vi "Draw ROI (user interactive).vi"(0 "Image file path":path) -> (1 "ROI to crop (pixels)":T1={"Xmax"=2147483647, "Ymax"=2147483647, "Xmin"=0, "Ymin"=0}, 2 "Error out":errorcluster)   [LabVIEW 2015]
doc: "Use this VI to mark a region-of-interest rectangle on an image, then programmatically output the ROI cluster and save the image with \"_ROI\" appended to current filename."
uses:
  Feature detection/Typedefs/ROI bounds.ctl
panel:
  in  "Quality":u32=750 max=1000
  out "Image showing ROI":T2(plugin-control)
  # "PN 04/04/2016"
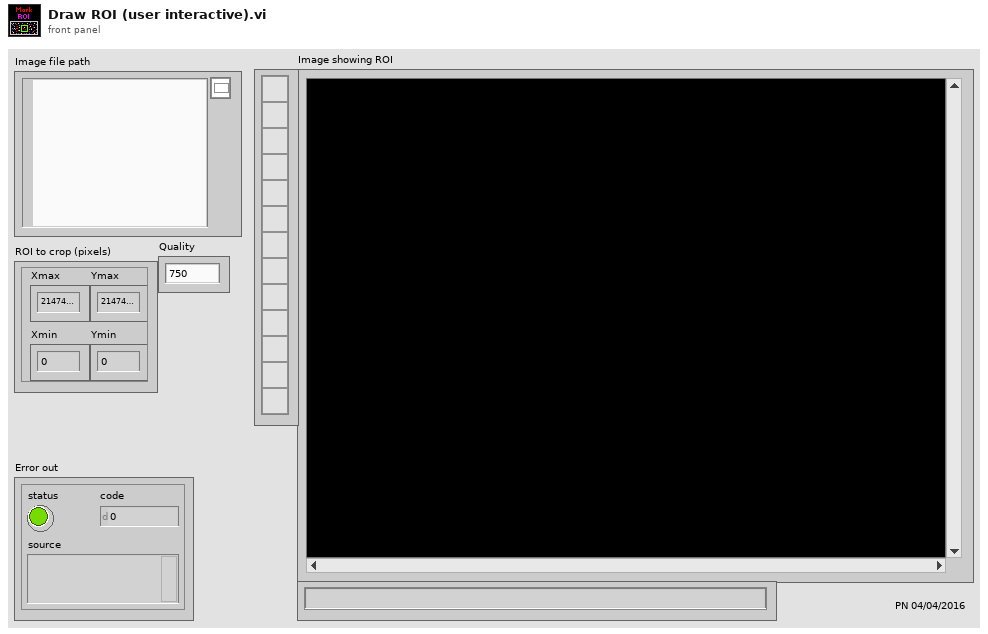
[diagram p1: front panel]
types:
  T1 = typedef "ROI bounds.ctl" = cluster{"Xmax":i32, "Ymax":i32, "Xmin":i32, "Ymin":i32}
  T2 = typedef "IMAQ Image.ctl" = refnum<image>
  T3 = cluster{"Left":i32, "Top":i32, "Right":i32, "Bottom":i32}
  T4 = typedef "Image Type" = u32
  T5 = typedef "IMAQ Rectangle" = cluster{"Left":i32, "Top":i32, "Right":i32, "Bottom":i32, "Rotation":dbl}
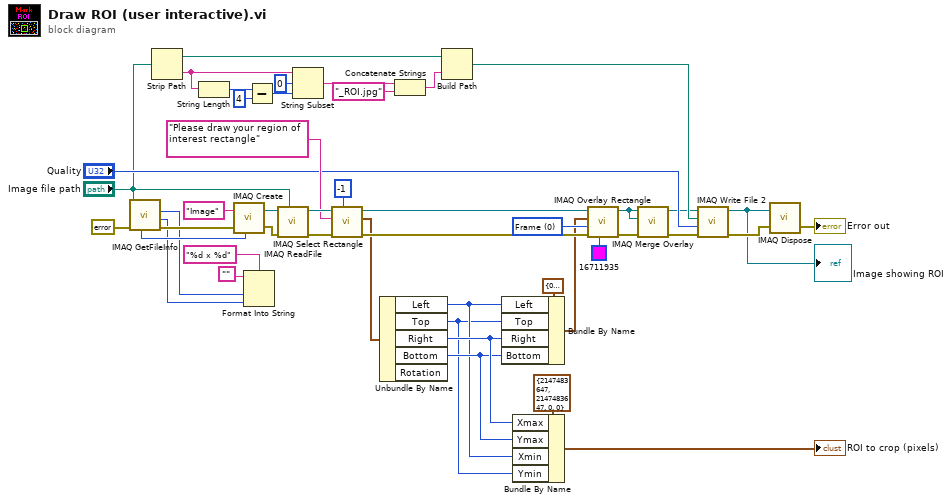
[diagram p0: block diagram]
diagram:
  w30 = u32 0 items=["Frame", "Fill", "Highlight"] ("Drawing Mode (Frame)")
  n1 = call "IMAQ GetFileInfo"("error in (no error)"=errorcluster {"status"=FALSE, "code"=0, "source"=""} ("error in"), "File Path"="Image file path") -> ("error out"=w41:errorcluster, "Y Resolution"=w39:i32, "X Resolution"=w40:i32, "Image Type"=w42:T4)  [unwired: 3 in, 3 out]
  n2 = Strip Path(path="Image file path") -> (stripped path=w14:path, name=w13:string)
  n3 = String Length(string=w13) -> (length=w12:i32)
  n4 = call "IMAQ Create"("Image Name"="Image", "Image Type"=w42, "error in (no error)"=w41) -> ("New Image"=w45:T2, "error out"=w44:errorcluster)  [unwired: 2 in]
  n5 = Format Into String(format string="%d x %d", initial string="", w40, w39) -> ()  [unwired: 1 in, 2 out]
  n6 = Subtract(x=w12, y=4) -> (x-y=w10:i32)
  n7 = call "IMAQ ReadFile"("File Path"="Image file path", "error in (no error)"=w44, "Image"=w45) -> ("error out"=w36:errorcluster, "Image Out"=w35:T2)  [unwired: 4 in, 3 out]
  n8 = String Subset(string=w13, offset (0)=0, length (rest)=w10) -> (substring=w8:string)
  n9 = call "IMAQ Select Rectangle"("Window Number (0...15)"=-1, "error in (no error)"=w36, "Prompt"="Please draw your region of interest rectangle", "Image In"=w35) -> ("error out"=w31:errorcluster, "Rectangle"=w29:T5, "Image Out (duplicate)"=w32:T2)  [unwired: 4 in, 1 out]
  n10 = Unbundle By Name(w29) -> ("Left"=w22:i32, "Top"=w21:i32, "Right"=w24:i32, "Bottom"=w23:i32)  [unwired: 1 out]
  n11 = Concatenate Strings(w8, "_ROI.jpg" ("string")) -> (w6:string)
  n12 = Build Path(base path=w14, name or relative path=w6) -> (appended path=w5:path)
  n13 = Bundle By Name(cluster=T3 {"Left"=0, "Top"=0, "Right"=0, "Bottom"=0} ("Rectangle"), "Left"=w22, "Top"=w21, "Right"=w24, "Bottom"=w23) -> (w27:T3)
  n14 = Bundle By Name(cluster=T1 {"Xmax"=2147483647, "Ymax"=2147483647, "Xmin"=0, "Ymin"=0} ("ROI to crop (pixels)"), "Xmax"=w24, "Ymax"=w23, "Xmin"=w22, "Ymin"=w21) -> (→"ROI to crop (pixels)":T1)
  n15 = call "IMAQ Overlay Rectangle"("Color"=u32 16711935, "error in (no error)"=w31, "Drawing Mode (Frame)"=w30, "Rectangle"=w27, "Image"=w32) -> ("error out"=w4:errorcluster, "Image Out"=w1:T2)  [unwired: 5 in]
  n16 = call "IMAQ Merge Overlay"("error in (no error)"=w4, "Image Dst"=w1, "Image Src"=w1) -> ("error out"=w2:errorcluster, "Image Dst Out"=w3:T2)  [unwired: 7 in]
  n17 = call-poly "IMAQ Write File 2"("error in (no error)"=w2, "Image Quality"="Quality", "File Path"=w5, "Image"=w3) -> ("error out"=w18:errorcluster, "Image Out (duplicate)"=w16:T2)  [unwired: 6 in]
  "Image showing ROI" <- w16
  n18 = call "IMAQ Dispose"("Image"=w16, "error in (no error)"=w18) -> ("error out"=→"Error out":errorcluster)  [unwired: 4 in]
